vi "Actor Core.vi"(8 "error in":errorcluster, 11 "RandomDataChart in":refnum<class "ActorAutoRegPanel.lvclass">) -> (0 "error out":errorcluster, 3 "Actor out":refnum<class "Actor.lvclass">)   [LabVIEW 2015, in "TestActors.lvlib" / "ActorAutoRegPanel.lvclass"]
doc: "(<B>Filename</B>: Actor Framework.lvlib:Actor.lvclass:Actor Core.vi)\n\nReceives messages to the actor, reacts to them, and initiates any error handling that may shut the actor down.\n\nDescendant classes may override this VI to append parallel tasks for the actor to complete while it handles messages. Overrides use the Call Parent Method node."
uses:
  ActorAutoRegPanel.lvclass
  <vilib>/ActorFramework/Actor/Actor.lvclass
  <vilib>/ActorFramework/Actor/Actor.lvclass/Actor.ctl
  <vilib>/ActorFramework/Message Enqueuer/Message Enqueuer.lvclass/Message Enqueuer.ctl
  <vilib>/ActorFramework/Message Enqueuer/Init from Existing Queue.vi
  IViewable/IViewable/IViewable.lvclass
  <vilib>/ActorFramework/Message Enqueuer/Message Enqueuer.lvclass
  AutoRegistration/ActorAutoRegistration/ActorAutoRegistration.lvclass
panel:
  in  "DBL":dbl
  in  "I32":i32
  in  "Whitaker":bool caption="Latch When Released"
  in  "Walton":bool caption="Latch Until Released"
  in  "Launch Dialog":bool
  in  "Guthrie":bool caption="Switch Until Released"
  in  "Harrelson":bool caption="Switch When Released"
  in  "Gump":bool caption="Latch When Pressed"
  in  "Wilson":bool caption="Switch When Pressed"
  # "An actor implementing\nfull auto-registration"
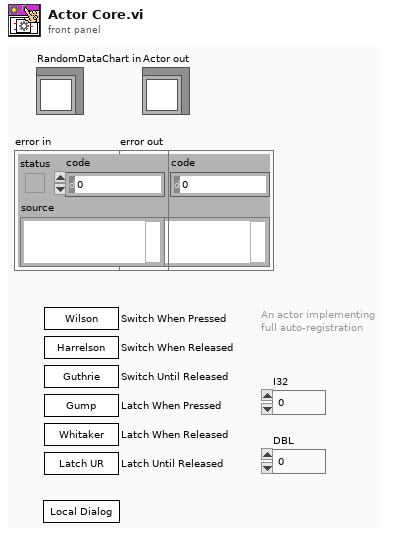
[diagram p1: front panel]
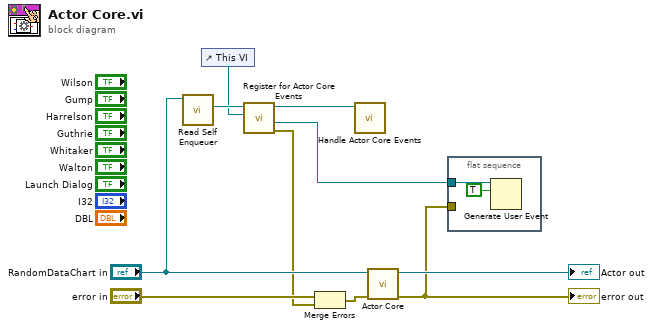
[diagram p0: block diagram]
diagram:
  n1 = call <vilib>:"Read Self Enqueuer.vi"("Actor"="RandomDataChart in") -> ("Self Enqueuer"=w3:refnum<class "Message Enqueuer.lvclass">)  [unwired: 10 in]
  n2 = control-ref of="This VI"() -> (w1:refnum<vi>)
  n3 = call "Register for Actor Core Events.vi"("VI Refnum (Actor Core)"=w1, "Actor Enqueuer"=w3) -> ("error out"=w4:errorcluster, "Stop! Event"=w6:refnum<user-event>, "ActorAutoRegistration Out"=w2:refnum<class "ActorAutoRegistration.lvclass">)  [unwired: 6 in, 1 out]
  n4 = Merge Errors("error in", w4) -> (w5:errorcluster)
  n5 = call-dynamic "Handle Actor Core Events.vi"("ActorAutoRegistration in"=w2) -> ()  [unwired: 9 in, 2 out]
  n6 = call-parent "Actor Core.vi"("error in"=w5, "IViewable In"="RandomDataChart in") -> ("error out"=w8:errorcluster, "Actor out"=→"Actor out":refnum<class "Actor.lvclass">)  [unwired: 8 in]
  "error out" <- w8
  n7 = flat-sequence {
    tunnel: w6 -> [w12]
    tunnel: w8 -> [_]
    frame #0 {
      n8 = Generate User Event(user event=w12, event data cluster=TRUE ("event data")) -> ()  [unwired: 2 in, 2 out]
    }
  }
